vi "Cmd Set Parameter Value (CR).vi"(6 "error in (no error)":errorcluster, 7 "value":variant, 8 "parameter index":variant, 9 "command-recordset reference":T1) -> (0 "error out":errorcluster, 3 "command-recordset reference out":T1)   [LabVIEW 2012, in "NI_Database_API_64.lvlib"]
doc: "Sets the value of the parameter at <B>parameter index</B> in the command or command-recordset. The <B>parameter index</B> can be either the zero-indexed position of the parameter in the command or the name of the parameter. Wire data to the reference input to determine the polymorphic instance to use or manually select the instance."
uses:
  NI_Database_API_64.lvlib
  Command-Recordset.llb/Cmd-Rec Object Reference.ctl
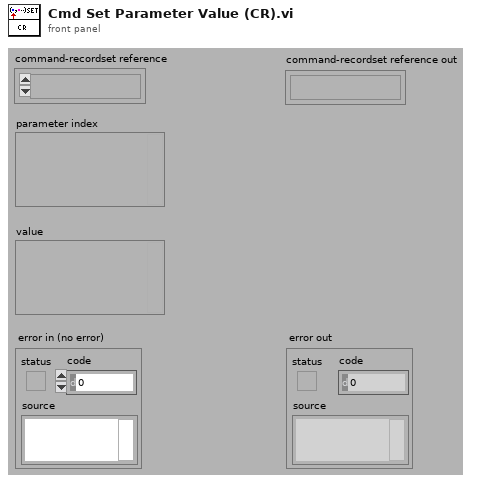
[diagram p1: front panel]
types:
  T1 = typedef "NI_Database_API_64.lvlib/Cmd-Rec Object Reference.ctl" = refnum<k1>
  T2 = typedef "NI_Database_API_64.lvlib/Cmd-Rec Data Members.ctl" = cluster{"recordset reference":T3, "command reference":T4}
  T3 = typedef "NI_Database_API_64.lvlib/Rec ObjectReference.ctl" = refnum<k1>
  T4 = typedef "NI_Database_API_64.lvlib/Cmd ObjectReference.ctl" = refnum<k1>
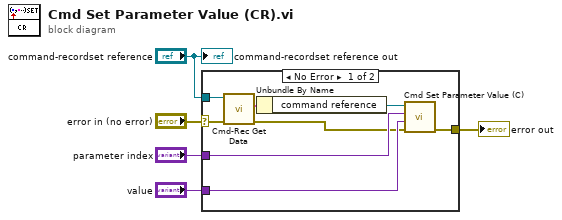
[diagram p0: block diagram]
diagram:
  n1 = case shown="No Error" "error in (no error)" {
    selector: "error in (no error)" -> [w6 w14]
    tunnel: "parameter index" -> [w13 _]
    tunnel: "value" -> [w12 _]
    tunnel: [w11 w14] -> w3
    tunnel: "command-recordset reference" -> [w7 _]
    frame No Error {
      n2 = call "Cmd-Rec Get Data.vi"("error in (no error)"=w6, "command-recordset reference"=w7) -> ("error out"=w8:errorcluster, "data"=w9:T2)  [unwired: 2 in, 2 out]
      n3 = Unbundle By Name(w9) -> ("command reference"=w10:T4)
      n4 = call "Cmd Set Parameter Value (C).vi"("error in (no error)"=w8, "value"=w12, "parameter index"=w13, "command reference"=w10) -> ("error out"=w11:errorcluster)  [unwired: 4 in, 1 out]
    }
    frame Error {
    }
  }
  "error out" <- w3
  "command-recordset reference out" <- "command-recordset reference"
